vi "数据处理.vi"() -> ()   [LabVIEW 2020]
uses:
  301c3acd-3236-4a35-8309-8f54d3b1edc5.vi
  <vilib>/Comparison/Less/Less Functor/Less Functor.lvclass
  viLib/QueueLib/QueueLib.lvlib
  viLib/LogLib/LogLib.lvlib
panel:
  in  "锁定突变电压":bool=TRUE
  out "数据属性":string[][](table)
  in  "索引簇":T1 {"下限" min=0; "上限" min=0; "索引" min=0}
  in  "拟合":bool
  in  "全部?":bool
  in  "包含删除？":T2
  in  "显示摘要":bool
  in  "测试类型":T3
  in  "显示曲线范围":T4=enum."Mixed"
  in  "删除":bool
  in  "打开数据":bool
  in  "数据显示":dbl[][](xcontrol)
  in  "导出数据选择":enum8{"False", "True", "Mixed"}(c332)
  in  "导出数据":bool
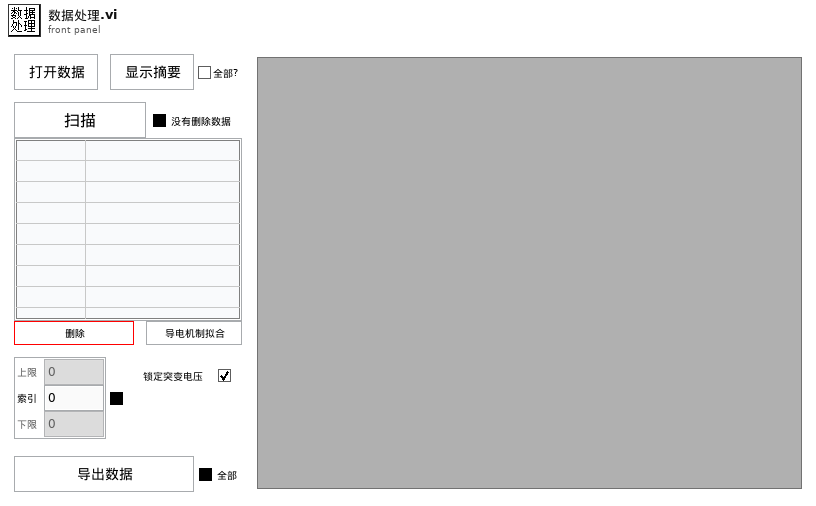
[diagram p1: front panel]
types:
  T1 = typedef "索引簇.ctl" = cluster{"上限":i32, "索引":i32, "下限":i32}
  T2 = typedef "包含删除.ctl" = enum8{"False", "True", "Mixed"}
  T3 = typedef "测试类型.ctl" = enum16{"扫描", "保持时间", "脉冲", "高速脉冲", "任意波形"}
  T4 = typedef "显示曲线范围.ctl" = enum8{"False", "True", "Mixed"}
  T5 = typedef "测试数据类型.ctl" = cluster{"测试时间":timestamp, "测试类型":string, "样品标记":string, "测试参数":variant, "循环":bool, "数据":dbl[][], "删除":bool, "突变电压":i32, "方向":string, "数据文件路径":path}
  T6 = typedef "QueueLib.lvlib/数据类型.ctl" = cluster{"消息":string, "数据":variant}
  T7 = enum8{"Enabled", "Disabled", "Disabled and Grayed Out"}
  T8 = typedef "数据类型.ctl" = cluster{"消息":string, "数据":variant}
  T9 = typedef "数据显示.xctl/波形数据定义.ctl" = cluster{"波形":dbl[][], "属性":variant}
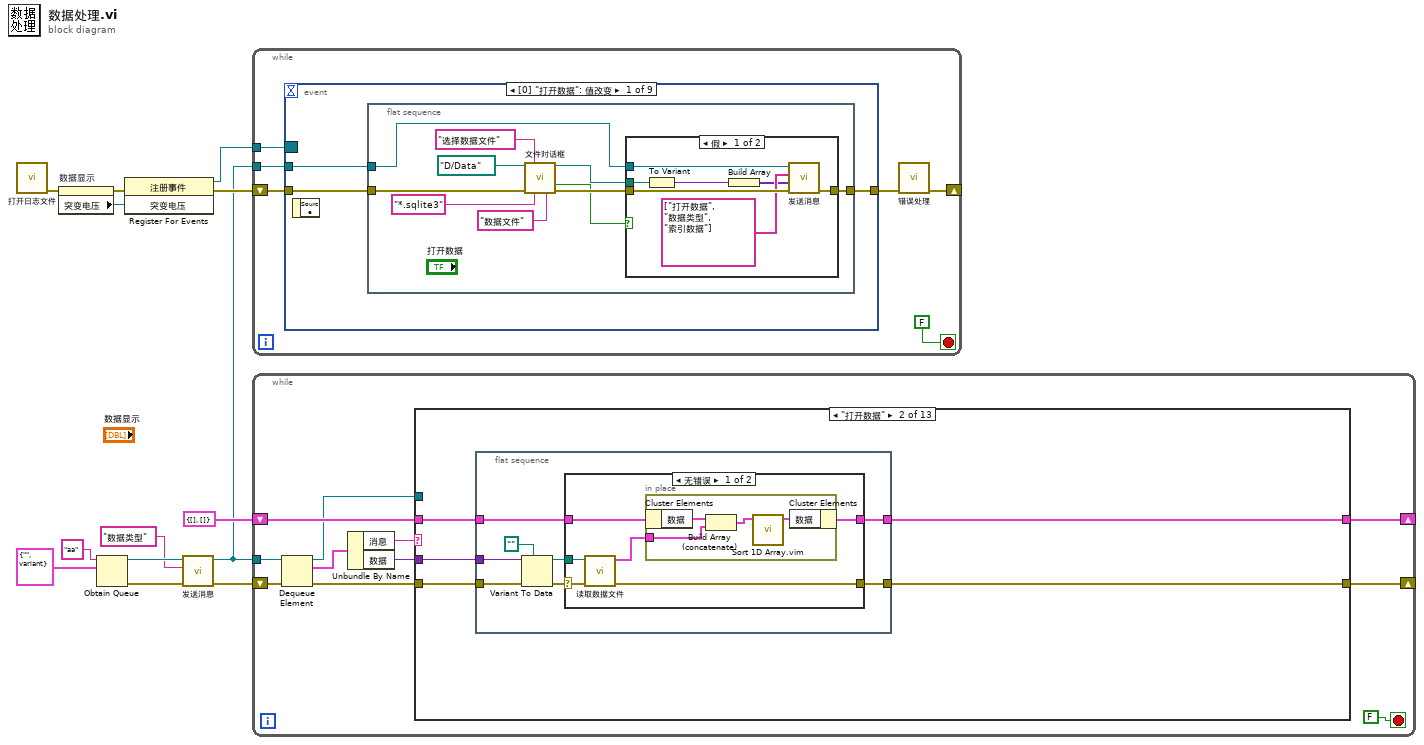
[diagram p0: block diagram]
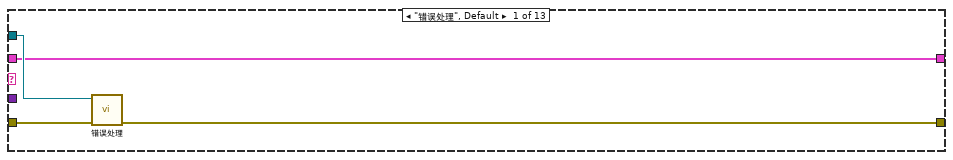
[diagram p2: hidden frame]
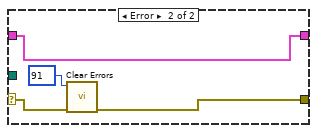
[diagram p3: hidden frame]
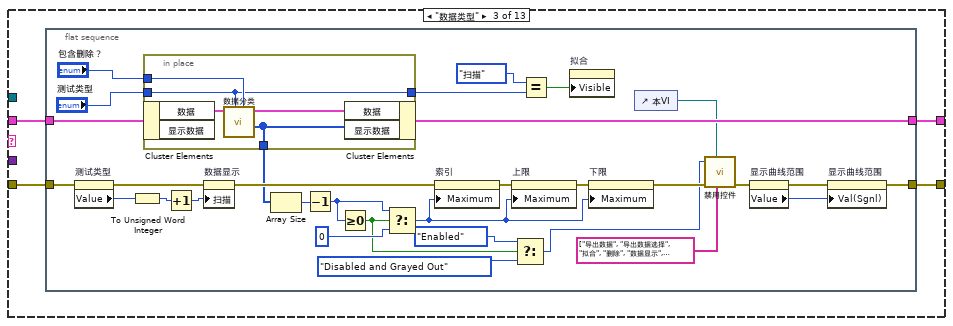
[diagram p4: hidden frame]
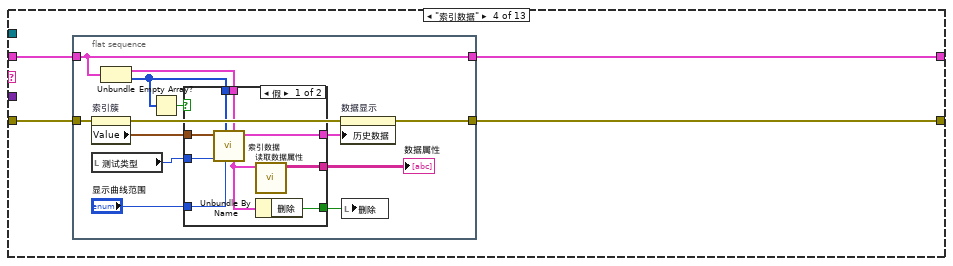
[diagram p5: hidden frame]
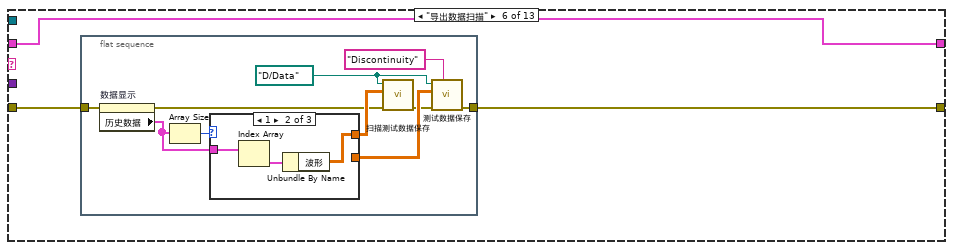
[diagram p8: hidden frame]
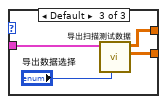
[diagram p10: hidden frame]
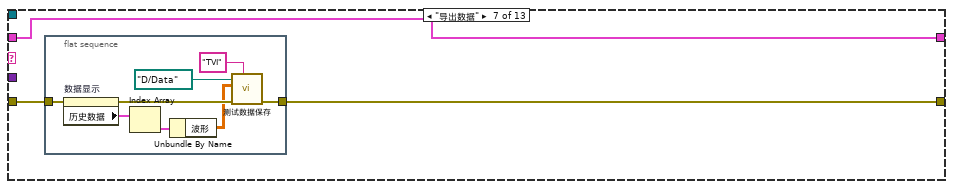
[diagram p11: hidden frame]
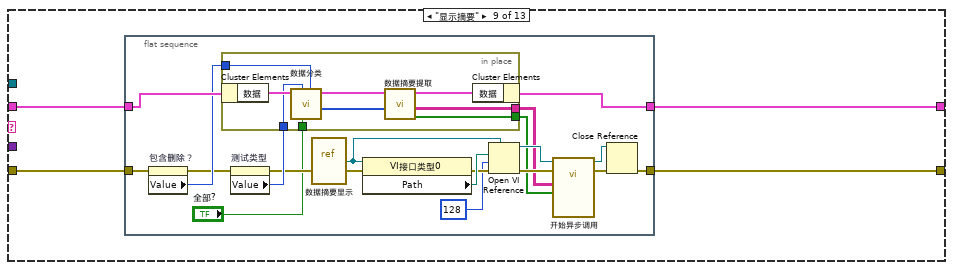
[diagram p13: hidden frame]
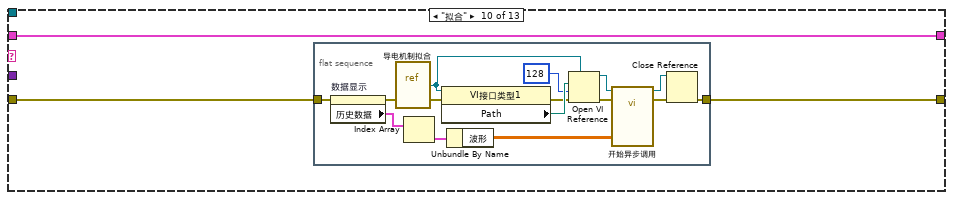
[diagram p14: hidden frame]
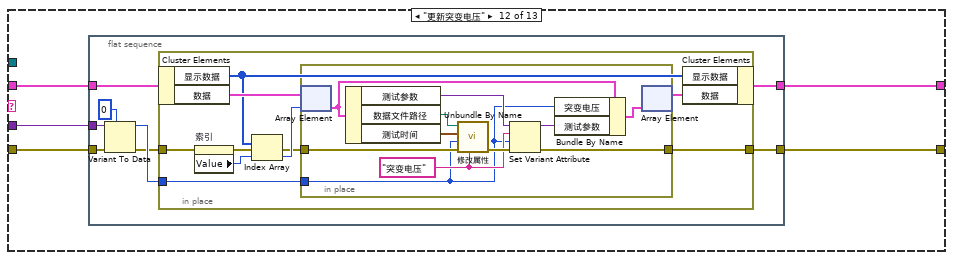
[diagram p16: hidden frame]
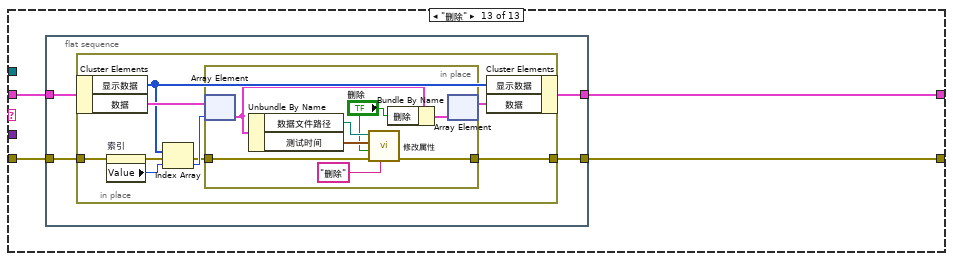
[diagram p17: hidden frame]
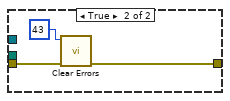
[diagram p18: hidden frame]
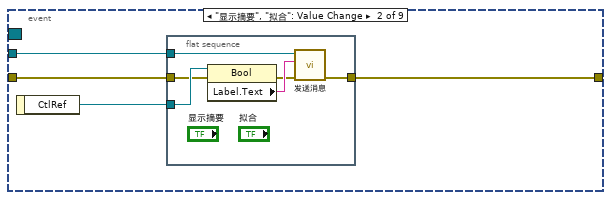
[diagram p19: hidden frame]
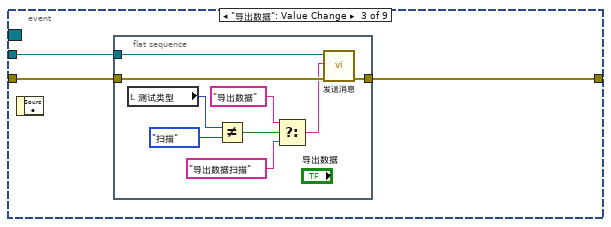
[diagram p20: hidden frame]
diagram:
  n1 = call "打开日志文件.vi"() -> ("错误输出"=w5:errorcluster)  [unwired: 11 in]
  n2 = property on="数据显示" class="数据显示 (严格)"(error in=w5) -> (error out=w6:errorcluster, "突变电压"=w9:refnum<user-event>)  [unwired: 1 in, 1 out]
  n3 = Obtain Queue(name (unnamed)="aa" ("名称（未命名）"), element data type=T6 {"消息"="", "数据"=variant} ("数据类型")) -> (queue out=w3:refnum<queue>, error out=w13:errorcluster)  [unwired: 3 in, 1 out]
  n4 = register-events(error in=w6, w9) -> (reference out=w8:refnum<event-registration>, error out=w7:errorcluster)  [unwired: 1 in]
  n5 = call-poly "发送消息.vi"("错误输入（无错误）"=w13, "消息"="数据类型", "输入队列"=w3) -> ("错误输出"=w4:errorcluster, "输出队列"=w2:refnum<queue>)  [unwired: 7 in]
  n6 = while {
    tunnel: w2 -> [w18]
    shift-right: [w16] -> _
    shift-left: w7 -> [w17]
    tunnel: w8 -> [w14]
    stop <- FALSE stop-if-true
    n7 = event shown="[0] \"打开数据\": 值改变" {
      selector: w14 -> [_ _ _ _ _ _ _ _ _]
      dyn-events: _ -> [_ _ _ _ _ _ _ _ _]
      timeout: _ -> [_ _ _ _ _ _ _ _ _]
      tunnel: w18 -> [w21 w45 w53 w68 w83 _ _ _ w142]
      tunnel: w17 -> [w20 w43 w55 w66 w81 w98 w119 w128 w141]
      tunnel: [w22 w46 w54 w67 w82 w97 w118 w127 w143] -> w15
      event "打开数据": Value Change {
        n8 = event-data() -> ()  [unwired: 1 in, 1 out]
        n9 = flat-sequence {
          tunnel: [w32] -> w22
          tunnel: w21 -> [w31]
          tunnel: w20 -> [w29]
          frame #0 {
            n10 = call "文件对话框"("start path"=path "D:/Data", "prompt"="选择数据文件", "error in"=w29, "pattern (all files)"="*.sqlite3", "pattern label"="数据文件") -> ("selected path"=w27:path, "cancelled"=w26:bool, "error out"=w28:errorcluster)  [unwired: 7 in, 1 out]
            n11 = case shown="假" w26 {
              tunnel: [w39 w41] -> w32
              tunnel: w31 -> [w38 _]
              tunnel: w28 -> [w37 w42]
              tunnel: w27 -> [w35 _]
              frame False {
                n12 = To Variant(anything=w35) -> (Variant=w34:variant)
                n13 = Build Array(w34) -> (w33:variant[])
                n14 = call-poly "发送消息.vi"("错误输入（无错误）"=w37, "数据列表"=w33, "消息列表"=string[] ["打开数据", "数据类型", "索引数据"], "输入队列"=w38) -> ("错误输出"=w39:errorcluster)  [unwired: 6 in, 1 out]
              }
              frame True {
                n15 = call <vilib>:"Clear Errors.vi"("error in (no error)"=w42, "specific error code to clear (0: all)"=43) -> ("error out"=w41:errorcluster)  [unwired: 4 in, 1 out]
              }
            }
          }
        }
      }
      event "显示摘要", "拟合": Value Change {
        n16 = event-data() -> ("CtlRef"=w44:refnum<vi>)  [unwired: 1 in]
        n17 = flat-sequence {
          tunnel: [w52] -> w46
          tunnel: w45 -> [w51]
          tunnel: w44 -> [w50]
          tunnel: w43 -> [w49]
          frame #0 {
            n18 = property class="Bool"(reference=w50, error in=w49) -> (error out=w47:errorcluster, "Label.Text"=w48:string)  [unwired: 1 out]
            n19 = call-poly "发送消息.vi"("错误输入（无错误）"=w47, "消息"=w48, "输入队列"=w51) -> ("错误输出"=w52:errorcluster)  [unwired: 7 in, 1 out]
          }
        }
      }
      event "导出数据": Value Change {
        n20 = event-data() -> ()  [unwired: 1 in, 1 out]
        n21 = flat-sequence {
          tunnel: [w64] -> w54
          tunnel: w53 -> [w63]
          tunnel: w55 -> [w62]
          frame #0 {
            n22 = local read "测试类型"() -> (w61:T3)
            n23 = Not Equal?(x=w61, y=测试类型."扫描") -> (x != y?=w59:bool)
            n24 = Select(t="导出数据", s=w59, f="导出数据扫描") -> (s? t:f=w56:string)
            n25 = call-poly "发送消息.vi"("错误输入（无错误）"=w62, "消息"=w56, "输入队列"=w63) -> ("错误输出"=w64:errorcluster)  [unwired: 7 in, 1 out]
          }
        }
      }
      event "删除": Value Change {
        n26 = event-data() -> ("CtlRef"=w65:refnum<vi>)  [unwired: 1 in]
        n27 = flat-sequence {
          tunnel: w68 -> [w79]
          tunnel: [w78] -> w67
          tunnel: w66 -> [w77]
          tunnel: w65 -> [w75]
          frame #0 {
            w73 = "删除" ("y")
            w72 = string[] ["数据类型", "索引数据"]
            n28 = property class="Ctl"(reference=w75, error in=w77) -> (error out=w76:errorcluster, "Label.Text"=w69:string)  [unwired: 1 out]
            n29 = Equal?(x=w69, y=w73) -> (x = y?=w74:bool)
            n30 = Build Array (concatenate)(w73, w72) -> (w71:string[])
            n31 = Select(t=w71, s=w74, f=w72) -> (s? t:f=w70:string[])
            n32 = call-poly "发送消息.vi"("错误输入（无错误）"=w76, "消息列表"=w70, "输入队列"=w79) -> ("错误输出"=w78:errorcluster)  [unwired: 7 in, 1 out]
          }
        }
      }
      event User Event {
        n33 = event-data() -> ("点索引"=w80:i32)  [unwired: 1 in]
        n34 = flat-sequence {
          tunnel: w83 -> [w88]
          tunnel: [w87] -> w82
          tunnel: w81 -> [w86]
          tunnel: w80 -> [w85]
          frame #0 {
            n35 = case shown="假" "锁定突变电压" {
              tunnel: w88 -> [w95 _]
              tunnel: [w93 w96] -> w87
              tunnel: w86 -> [w92 w96]
              tunnel: w85 -> [w91 _]
              frame False {
                n36 = To Variant(anything=w91) -> (Variant=w90:variant)
                n37 = Build Array(w90) -> (w89:variant[])
                n38 = call-poly "发送消息.vi"("错误输入（无错误）"=w92, "数据列表"=w89, "消息列表"=string[] ["更新突变电压", "索引数据"], "输入队列"=w95) -> ("错误输出"=w93:errorcluster)  [unwired: 6 in, 1 out]
              }
              frame True {
              }
            }
          }
        }
      }
      event Key Down {
        n39 = event-data() -> ("ScanCode"=w99:i16)  [unwired: 1 in]
        n40 = flat-sequence {
          tunnel: w99 -> [w102]
          tunnel: w98 -> [w101]
          tunnel: [w100] -> w97
          frame #0 {
            n41 = case shown="72, 80" w102 {
              selector: w102 -> [_ w105 _]
              tunnel: w101 -> [w103 w109 w116]
              tunnel: [w103 w107 w115] -> w100
              frame 0, Default {
              }
              frame 72, 80 {
                n42 = property on="索引" class="DigNum (严格)"(error in=w109) -> (error out=w108:errorcluster, "Value"=w106:i32)  [unwired: 1 in, 1 out]
                n43 = case shown="72" w105 {
                  tunnel: w106 -> [w111 w113]
                  tunnel: [w110 w112] -> w104
                  frame Default {
                    n44 = Decrement(x=w111) -> (x-1=w110:i32)
                  }
                  frame 72 {
                    n45 = Increment(x=w113) -> (x+1=w112:i32)
                  }
                }
                n46 = property on="索引" class="DigNum (严格)"(error in=w108, "Val(Sgnl)"=w104) -> (error out=w107:errorcluster)  [unwired: 1 in, 1 out]
              }
              frame 83 {
                n47 = property on="删除" class="Bool (严格)"(error in=w116, "Val(Sgnl)"=TRUE ("值(信号)")) -> (error out=w115:errorcluster)  [unwired: 1 in, 1 out]
              }
            }
          }
        }
      }
      event Mouse Wheel {
        n48 = event-data() -> ("Delta"=w117:i32)  [unwired: 1 in]
        n49 = flat-sequence {
          tunnel: w119 -> [w125]
          tunnel: [w124] -> w118
          tunnel: w117 -> [w121]
          frame #0 {
            n50 = property on="索引" class="DigNum (严格)"(error in=w125) -> (error out=w123:errorcluster, "Value"=w120:i32)  [unwired: 1 in, 1 out]
            n51 = Add(x=w120, y=w121) -> (x+y=w122:i32)
            n52 = property on="索引" class="DigNum (严格)"(error in=w123, "Val(Sgnl)"=w122) -> (error out=w124:errorcluster)  [unwired: 1 in, 1 out]
          }
        }
      }
      event Value Change {
        n53 = event-data() -> ("NewVal"=w126:T4)  [unwired: 1 in]
        n54 = flat-sequence {
          tunnel: w128 -> [w140]
          tunnel: [w139] -> w127
          tunnel: w126 -> [w138]
          frame #0 {
            n55 = Equal?(x=w138, y=enum8{"False", "True", "Mixed"}."True") -> (x = y?=w136:bool)
            n56 = property on="上限" class="DigNum (严格)"(error in=w140) -> (error out=w131:errorcluster, "Maximum"=w130:dbl)  [unwired: 1 in, 1 out]
            n57 = Select(t=T7."Enabled" ("禁用"), s=w136, f=T7."Disabled and Grayed Out") -> (s? t:f=w133:T7)
            n58 = property on="上限" class="DigNum (严格)"(error in=w131, "Value"=w130, "DisabledEnum"=w133) -> (error out=w132:errorcluster, "Minimum"=w129:dbl)  [unwired: 1 in, 1 out]
            n59 = property on="下限" class="DigNum (严格)"(error in=w132, "Val(Sgnl)"=w129, "DisabledEnum"=w133) -> (error out=w139:errorcluster)  [unwired: 1 in, 1 out]
          }
        }
      }
      event Value Change {
        n60 = event-data() -> ()  [unwired: 1 in, 1 out]
        n61 = flat-sequence {
          tunnel: [w153] -> w143
          tunnel: w142 -> [w152]
          tunnel: w141 -> [w149]
          frame #0 {
            n62 = Unbundle By Name("索引簇") -> ("上限"=w146:i32, "索引"=w145:i32, "下限"=w144:i32)
            n63 = In Range and Coerce(upper limit=w146, x=w145, lower limit=w144) -> (coerced(x)=w151:i32, In Range?=w148:bool)
            n64 = property on="索引" class="DigNum (严格)"(error in=w149, "Value"=w151) -> (error out=w150:errorcluster)  [unwired: 1 in, 1 out]
            n65 = case shown="真" w148 {
              tunnel: w150 -> [w154 w158]
              tunnel: w152 -> [_ w157]
              tunnel: [w154 w156] -> w153
              frame False {
              }
              frame True {
                n66 = call-poly "发送消息.vi"("错误输入（无错误）"=w158, "消息"="索引数据", "输入队列"=w157) -> ("错误输出"=w156:errorcluster)  [unwired: 7 in, 1 out]
              }
            }
          }
        }
      }
    }
    n67 = call "错误处理.vi"("错误输入（无错误）"=w15) -> ("错误输出"=w16:errorcluster)  [unwired: 9 in, 1 out]
  }
  n68 = while {
    tunnel: w2 -> [w169]
    shift-right: [w160] -> _
    shift-left: w4 -> [w168]
    shift-right: [w159] -> _
    shift-left: cluster{"数据":T5[], "显示数据":i32[]} {"数据"=[], "显示数据"=[]} -> [w164]
    stop <- FALSE stop-if-true
    n69 = Dequeue Element(queue=w169, error in (no error)=w168) -> (queue out=w161:refnum<queue>, element=w166:T8, error out=w167:errorcluster)  [unwired: 1 in, 1 out]
    n70 = Unbundle By Name(w166) -> ("消息"=w165:string, "数据"=w162:variant)
    n71 = case shown="\"打开数据\"" w165 {
      tunnel: w167 -> [w173 w178 w203 w243 w268 w269 w289 w301 w304 w334 w352 w357 w389]
      tunnel: [w172 w174 w201 w242 w268 w270 w290 w301 w305 w335 w352 w353 w388] -> w160
      tunnel: [w170 w175 w202 w241 w267 w271 w291 w300 w303 w336 w351 w354 w386] -> w159
      tunnel: w164 -> [w170 w176 w204 w244 w267 w271 w291 w300 w302 w336 w351 w356 w387]
      tunnel: w162 -> [_ w177 _ _ _ _ _ _ _ _ _ w355 _]
      tunnel: w161 -> [w171 _ _ _ _ _ _ _ _ _ _ _ _]
      frame "错误处理", Default {
        n72 = call "错误处理.vi"("错误输入（无错误）"=w173, "队列输入"=w171) -> ("错误输出"=w172:errorcluster)  [unwired: 8 in, 1 out]
      }
      frame "打开数据" {
        n73 = flat-sequence {
          tunnel: w178 -> [w186]
          tunnel: w177 -> [w185]
          tunnel: w176 -> [w184]
          tunnel: [w180] -> w175
          tunnel: [w179] -> w174
          frame #0 {
            n74 = Variant To Data(error in=w186, type=path "", Variant=w185) -> (data=w182:path, error out=w181:errorcluster)
            n75 = case shown="无错误" w181 {
              selector: w181 -> [w190 w200]
              tunnel: [w192 w199] -> w179
              tunnel: w184 -> [w189 w197]
              tunnel: [w188 w197] -> w180
              tunnel: w182 -> [w191 _]
              frame No Error {
                n76 = call "读取数据文件.vi"("错误输入（无错误）"=w190, "数据文件路径"=w191) -> ("错误输出"=w192:errorcluster, "数据"=w187:T5[])  [unwired: 8 in]
                n77 = in-place {
                  in-place-border: w187 -> [w195]
                  n78 = in-place-cluster #1(w189) -> ("数据"=w196:T5[])
                  n79 = Build Array (concatenate)(w196, w195) -> (w194:T5[])
                  n80 = call "Sort 1D Array.vim"("unsorted array"=w194) -> ("sorted array"=w193:T5[])  [unwired: 10 in]
                  n81 = in-place-cluster #1("数据"=w193) -> (w188:cluster{"数据":T5[], "显示数据":i32[]})
                }
              }
              frame Error {
                n82 = call <vilib>:"Clear Errors.vi"("error in (no error)"=w200, "specific error code to clear (0: all)"=91) -> ("error out"=w199:errorcluster)  [unwired: 4 in, 1 out]
              }
            }
          }
        }
      }
      frame "数据类型" {
        n83 = flat-sequence {
          tunnel: w204 -> [w235]
          tunnel: w203 -> [w225]
          tunnel: [w232] -> w202
          tunnel: [w223] -> w201
          frame #0 {
            n84 = property on="测试类型" class="Enum (严格)"(error in=w225) -> (error out=w226:errorcluster, "Value"=w229:T3)  [unwired: 1 in, 1 out]
            n85 = To Unsigned Word Integer(number=w229) -> (unsigned 16bit integer=w228:u16)
            n86 = in-place {
              in-place-border: "测试类型" -> [w236]
              in-place-border: "包含删除？" -> [w238]
              in-place-border: [w237] -> w219
              in-place-border: [w236] -> w206
              n87 = in-place-cluster #2(w235) -> ("数据"=w240:T5[])  [unwired: 1 out]
              n88 = call "数据分类.vi"("包含删除？"=w238, "测试类型"=w236, "数组输入"=w240) -> ("数据索引"=w237:i32[], "数组输出"=w239:T5[])  [unwired: 7 in]
              n89 = in-place-cluster #2("数据"=w239, "显示数据"=w237) -> (w232:cluster{"数据":T5[], "显示数据":i32[]})
            }
            n90 = Increment(x=w228) -> (x+1=w227:u16)
            n91 = property on="数据显示" class="数据显示 (严格)"(error in=w226, "扫描"=w227) -> (error out=w224:errorcluster)  [unwired: 1 in, 1 out]
            n92 = Array Size(array=w219) -> (size(s)=w220:i32)
            n93 = Decrement(x=w220) -> (x-1=w217:i32)
            n94 = Greater Or Equal To 0?(x=w217) -> (x >= 0?=w209:bool)
            n95 = Select(t=w217, s=w209, f=0) -> (s? t:f=w218:i32)
            n96 = property on="索引" class="DigNum (严格)"(error in=w224, "Maximum"=w218) -> (error out=w231:errorcluster)  [unwired: 1 in, 1 out]
            n97 = property on="上限" class="DigNum (严格)"(error in=w231, "Maximum"=w218) -> (error out=w230:errorcluster)  [unwired: 1 in, 1 out]
            n98 = Select(t=T7."Enabled" ("禁用"), s=w209, f=T7."Disabled and Grayed Out") -> (s? t:f=w211:T7)
            n99 = Equal?(x=测试类型."扫描", y=w206) -> (x = y?=w207:bool)
            n100 = property on="拟合" class="Bool"("Visible"=w207) -> ()  [unwired: 2 in, 2 out]
            n101 = property on="下限" class="DigNum (严格)"(error in=w230, "Maximum"=w218) -> (error out=w214:errorcluster)  [unwired: 1 in, 1 out]
            n102 = control-ref of="本VI"() -> (w215:refnum<vi>)
            n103 = call "禁用控件.vi"("控件名称"=string[] ["导出数据", "导出数据选择", "拟合", "删除", "数据显示", "数据属性", "索引簇", "显示曲线范围"], "本VI"=w215, "错误输入（无错误）"=w214, "禁用"=w211) -> ("错误输出"=w213:errorcluster)  [unwired: 7 in]
            n104 = property on="显示曲线范围" class="MixedCheckbox (严格)"(error in=w213) -> (error out=w222:errorcluster, "Value"=w221:T4)  [unwired: 1 in, 1 out]
            n105 = property on="显示曲线范围" class="MixedCheckbox (严格)"(error in=w222, "Val(Sgnl)"=w221) -> (error out=w223:errorcluster)  [unwired: 1 in, 1 out]
          }
        }
      }
      frame "索引数据" {
        n106 = flat-sequence {
          tunnel: w244 -> [w248]
          tunnel: w243 -> [w256]
          tunnel: [w254] -> w242
          tunnel: [w248] -> w241
          frame #0 {
            n107 = property on="索引簇" class="Clust (严格)"(error in=w256) -> (error out=w255:errorcluster, "Value"=w252:T1)  [unwired: 1 in, 1 out]
            n108 = local read "测试类型"() -> (w245:T3)
            n109 = Unbundle(w248) -> ("数据"=w253:T5[], "显示数据"=w246:i32[])
            n110 = Empty Array?(array=w246) -> (empty?=w247:bool)
            n111 = case shown="假" w247 {
              tunnel: [w266 _] -> w257
              tunnel: w246 -> [w265 _]
              tunnel: w253 -> [w264 _]
              tunnel: w252 -> [w263 _]
              tunnel: [w262 _] -> w251
              tunnel: "显示曲线范围" -> [w261 _]
              tunnel: [w259 _] -> w249
              tunnel: w245 -> [w258 _]
              frame False {
                n112 = call "索引数据.vi"("数据"=w264, "显示曲线范围"=w261, "显示数据"=w265, "测试类型"=w258, "索引簇"=w263) -> ("数组"=w266:T9[], "当前索引"=w260:T5)  [unwired: 5 in]
                n113 = call "读取数据属性.vi"("测试数据"=w260) -> ("数据属性"=w262:string[][])  [unwired: 10 in]
                n114 = Unbundle By Name(w260) -> ("删除"=w259:bool)
              }
              frame True {
              }
            }
            "数据属性" <- w251
            n115 = property on="数据显示" class="数据显示 (严格)"(error in=w255, "历史数据"=w257) -> (error out=w254:errorcluster)  [unwired: 1 in, 1 out]
            n116 = local write "删除"(w249) -> ()
          }
        }
      }
      frame "==== 导出 ====" {
      }
      frame "导出数据扫描" {
        n117 = flat-sequence {
          tunnel: [w281] -> w270
          tunnel: w269 -> [w278]
          frame #0 {
            w275 = path "D:/Data" ("start path")
            n118 = property on="数据显示" class="数据显示 (严格)"(error in=w278) -> (error out=w277:errorcluster, "历史数据"=w274:T9[])  [unwired: 1 in, 1 out]
            n119 = Array Size(array=w274) -> (size(s)=w273:i32)
            n120 = case shown="1" w273 {
              tunnel: w274 -> [_ w284 w288]
              tunnel: [_ w282 w286] -> w280
              tunnel: [_ _ w285] -> w279
              frame 0 {
              }
              frame 1 {
                n121 = Index Array(array=w284) -> (element=w283:T9)  [unwired: 1 in]
                n122 = Unbundle By Name(w283) -> ("波形"=w282:dbl[][])
              }
              frame Default {
                n123 = call "导出扫描测试数据.vi"("导出数据选择"="导出数据选择", "数据"=w288) -> ("突变电压"=w285:dbl[][], "扫描数据"=w286:dbl[][])  [unwired: 8 in]
              }
            }
            n124 = call "扫描测试数据保存.vi"("错误输入（无错误）"=w277, "扫描数据"=w280, "start path"=w275) -> ("错误输出"=w276:errorcluster)  [unwired: 8 in]
            n125 = call "测试数据保存.vi"("文件名称前缀"="Discontinuity", "错误输入（无错误）"=w276, "数据"=w279, "start path"=w275) -> ("错误输出"=w281:errorcluster)  [unwired: 7 in]
          }
        }
      }
      frame "导出数据" {
        n126 = flat-sequence {
          tunnel: [w299] -> w290
          tunnel: w289 -> [w298]
          frame #0 {
            n127 = property on="数据显示" class="数据显示 (严格)"(error in=w298) -> (error out=w297:errorcluster, "历史数据"=w296:T9[])  [unwired: 1 in, 1 out]
            n128 = Index Array(array=w296) -> (element=w295:T9)  [unwired: 1 in]
            n129 = Unbundle By Name(w295) -> ("波形"=w294:dbl[][])
            n130 = call "测试数据保存.vi"("文件名称前缀"="TVI", "错误输入（无错误）"=w297, "数据"=w294, "start path"=path "D:/Data") -> ("错误输出"=w299:errorcluster)  [unwired: 7 in]
          }
        }
      }
      frame "==== 数据展示 ====" {
      }
      frame "显示摘要" {
        n131 = flat-sequence {
          tunnel: [w306] -> w305
          tunnel: w304 -> [w311]
          tunnel: [w324] -> w303
          tunnel: w302 -> [w323]
          frame #0 {
            n132 = property on="包含删除？" class="MixedCheckbox (严格)"(error in=w311) -> (error out=w310:errorcluster, "Value"=w312:T2)  [unwired: 1 in, 1 out]
            n133 = property on="测试类型" class="Enum (严格)"(error in=w310) -> (error out=w309:errorcluster, "Value"=w313:T3)  [unwired: 1 in, 1 out]
            n134 = in-place {
              in-place-border: [w332] -> w315
              in-place-border: [w331] -> w314
              in-place-border: w313 -> [w328]
              in-place-border: w312 -> [w327]
              in-place-border: "全部?" -> [w326]
              n135 = in-place-cluster #3(w323) -> ("数据"=w330:T5[])
              n136 = call "数据分类.vi"("包含删除？"=w327, "所有类型"=w326, "测试类型"=w328, "数组输入"=w330) -> ("数据索引"=w325:i32[], "数组输出"=w333:T5[])  [unwired: 6 in]
              n137 = call "数据摘要提取.vi"("数据索引"=w325, "数组输入"=w333) -> ("删除？"=w332:bool[], "数据摘要"=w331:string[][], "数组输出"=w329:T5[])  [unwired: 7 in]
              n138 = in-place-cluster #3("数据"=w329) -> (w324:cluster{"数据":T5[], "显示数据":i32[]})
            }
            n139 = vi-ref "数据摘要显示.vi"() -> (w318:refnum<vi>)
            n140 = property class="VI接口类型0"(reference=w318, error in=w309) -> (error out=w316:errorcluster, "Path"=w317:path)  [unwired: 1 out]
            n141 = Open VI Reference(type specifier VI Refnum (for type only)=w318, vi path=w317, options=128 ("选项"), error in (no error)=w316) -> (vi reference=w322:refnum<vi>, error out=w321:errorcluster)  [unwired: 2 in]
            n142 = call-by-ref "开始异步调用"(reference=w322, error in=w321, "删除？"=w315, "数据摘要"=w314) -> (reference out=w320:refnum<vi>, error out=w319:errorcluster)  [unwired: 10 in]
            n143 = Close Reference(reference=w320, error in (no error)=w319) -> (error out=w306:errorcluster)
          }
        }
      }
      frame "拟合" {
        n144 = flat-sequence {
          tunnel: [w338] -> w335
          tunnel: w334 -> [w343]
          frame #0 {
            n145 = property on="数据显示" class="数据显示 (严格)"(error in=w343) -> (error out=w342:errorcluster, "历史数据"=w341:T9[])  [unwired: 1 in, 1 out]
            n146 = vi-ref "导电机制拟合.vi"() -> (w350:refnum<vi>)
            n147 = Index Array(array=w341) -> (element=w340:T9)  [unwired: 1 in]
            n148 = property class="VI接口类型1"(reference=w350, error in=w342) -> (error out=w348:errorcluster, "Path"=w349:path)  [unwired: 1 out]
            n149 = Unbundle By Name(w340) -> ("波形"=w339:dbl[][])
            n150 = Open VI Reference(type specifier VI Refnum (for type only)=w350, vi path=w349, options=128 ("选项"), error in (no error)=w348) -> (vi reference=w346:refnum<vi>, error out=w345:errorcluster)  [unwired: 2 in]
            n151 = call-by-ref "开始异步调用"(reference=w346, error in=w345, "数据"=w339) -> (reference out=w337:refnum<vi>, error out=w344:errorcluster)  [unwired: 11 in]
            n152 = Close Reference(reference=w337, error in (no error)=w344) -> (error out=w338:errorcluster)
          }
        }
      }
      frame "==== 数据修改 ====" {
      }
      frame "更新突变电压" {
        n153 = flat-sequence {
          tunnel: w357 -> [w358]
          tunnel: w356 -> [w365]
          tunnel: w355 -> [w364]
          tunnel: [w361] -> w354
          tunnel: [w359] -> w353
          frame #0 {
            n154 = Variant To Data(error in=w358, type=0, Variant=w364) -> (data=w362:i32, error out=w360:errorcluster)
            n155 = in-place {
              in-place-border: w362 -> [w374]
              in-place-border: w360 -> [w367]
              in-place-border: [w373] -> w359
              n156 = in-place-cluster #4(w365) -> ("显示数据"=w370:i32[], "数据"=w372:T5[])
              n157 = property on="索引" class="DigNum (严格)"(error in=w367) -> (error out=w366:errorcluster, "Value"=w368:i32)  [unwired: 1 in, 1 out]
              n158 = Index Array(array=w370, index=w368) -> (element=w369:i32)
              n159 = in-place {
                in-place-border: w374 -> [w375]
                in-place-border: w366 -> [w380]
                in-place-border: [w384] -> w373
                w378 = "突变电压" ("属性名称")
                n160 = in-place-array #5(w372, w369) -> (w385:T5)
                n161 = Unbundle By Name(w385) -> ("测试参数"=w383:variant, "数据文件路径"=w377:path, "测试时间"=w376:timestamp)
                n162 = call "修改属性.vi"("属性名称"=w378, "错误输入（无错误）"=w380, "属性值"=w375, "测试时间"=w376, "db file"=w377) -> ("错误输出"=w379:errorcluster)  [unwired: 6 in]
                n163 = Set Variant Attribute(Variant=w383, name=w378, value=w375, error in=w379) -> (Variant out=w381:variant, error out=w384:errorcluster)  [unwired: 1 out]
                n164 = Bundle By Name(cluster=w385, "突变电压"=w375, "测试参数"=w381) -> (w382:T5)
                n165 = in-place-array #5(w382) -> (w371:T5[])  [unwired: 1 out]
              }
              n166 = in-place-cluster #4("显示数据"=w370, "数据"=w371) -> (w361:cluster{"数据":T5[], "显示数据":i32[]})
            }
          }
        }
      }
      frame "删除" {
        n167 = flat-sequence {
          tunnel: w389 -> [w390]
          tunnel: [w393] -> w388
          tunnel: w387 -> [w392]
          tunnel: [w391] -> w386
          frame #0 {
            n168 = in-place {
              in-place-border: [w394] -> w393
              in-place-border: w390 -> [w395]
              n169 = in-place-cluster #6(w392) -> ("显示数据"=w399:i32[], "数据"=w401:T5[])
              n170 = property on="索引" class="DigNum (严格)"(error in=w395) -> (error out=w397:errorcluster, "Value"=w396:i32)  [unwired: 1 in, 1 out]
              n171 = Index Array(array=w399, index=w396) -> (element=w398:i32)
              n172 = in-place {
                in-place-border: w397 -> [w407]
                in-place-border: [w406] -> w394
                n173 = in-place-array #7(w401, w398) -> (w409:T5)
                n174 = Unbundle By Name(w409) -> ("数据文件路径"=w403:path, "测试时间"=w404:timestamp)
                n175 = call "修改属性.vi"("属性名称"="删除", "错误输入（无错误）"=w407, "属性值"="删除", "测试时间"=w404, "db file"=w403) -> ("错误输出"=w406:errorcluster)  [unwired: 6 in]
                n176 = Bundle By Name(cluster=w409, "删除"="删除") -> (w408:T5)
                n177 = in-place-array #7(w408) -> (w400:T5[])  [unwired: 1 out]
              }
              n178 = in-place-cluster #6("显示数据"=w399, "数据"=w400) -> (w391:cluster{"数据":T5[], "显示数据":i32[]})
            }
          }
        }
      }
    }
  }
